vi "update_position.vi"(8 "error in (no error)":errorcluster, 11 "MH100301DMC in":refnum<class "StageMH100301DMC.lvclass">) -> (0 "error out":errorcluster, 3 "MH100301DMC out":refnum<class "StageMH100301DMC.lvclass">)   [LabVIEW 2010, in "StageMH100301DMC.lvclass"]
uses:
  StageMH100301DMC.lvclass
  StageDL090409Scaffold/StageDL090409Scaffold/StageDL090409Scaffold.lvclass
  common/classes/ErrorController/ErrorController/class_data.vi
  common/classes/ErrorController/ErrorController/ErrorController.lvclass
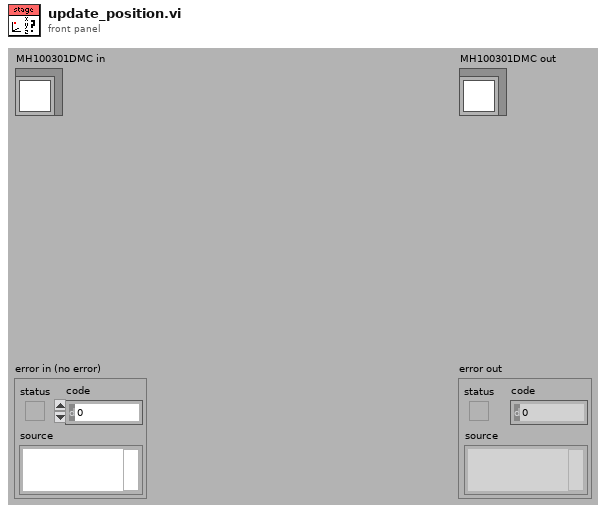
[diagram p1: front panel]
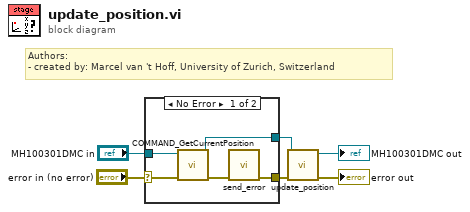
[diagram p0: block diagram]
diagram:
  # "Authors: \n- created by: Marcel van 't Hoff, University of Zurich, Switzerland"
  n1 = case shown="No Error" "error in (no error)" {
    selector: "error in (no error)" -> [w10 w13]
    tunnel: [w7 w13] -> w2
    tunnel: [w11 w12] -> w1
    tunnel: "MH100301DMC in" -> [w9 w12]
    frame No Error {
      n2 = call-dynamic "COMMAND_GetCurrentPosition.vi"("error in (no error)"=w10, "MH100301DMC in"=w9) -> ("error out"=w8:errorcluster, "MH100301DMC out"=w11:refnum<class "StageMH100301DMC.lvclass">)  [unwired: 7 in, 1 out]
      n3 = call "send_error.vi"("error in (no error)"=w8) -> ("error out"=w7:errorcluster)  [unwired: 10 in]
    }
    frame Error {
    }
  }
  n4 = call-parent "update_position.vi"("error in (no error)"=w2, "DL090409StageScaffold in"=w1) -> ("error out"=→"error out":errorcluster, "DL090409StageScaffold out"=→"MH100301DMC out":refnum<class "StageMH100301DMC.lvclass">)  [unwired: 8 in]
